vi "Destroy.vi"(8 "error in (no error)":errorcluster, 11 "reference in":refnum<class "Character.lvclass">) -> (0 "error out":errorcluster, 3 "reference out":refnum<class "Character.lvclass">)   [LabVIEW 2012, in "Character.lvclass"]
uses:
  Character.lvclass
  Glyph_class/Glyph.lvclass
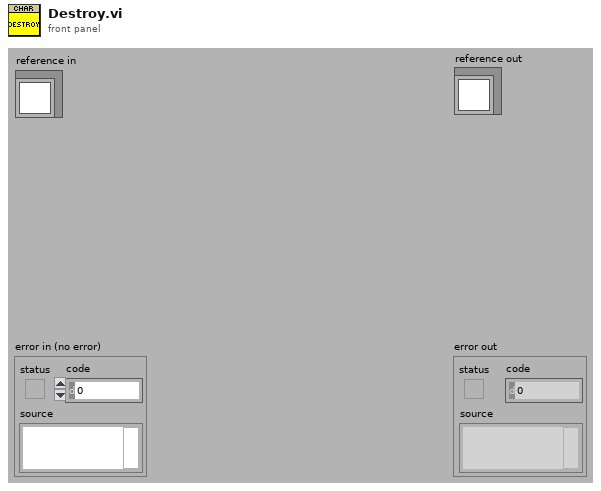
[diagram p1: front panel]
types:
  T1 = typedef "Character.lvclass/ObjectAttributes.ctl" = cluster{"Font":cluster{"Font Name:":string, "Size":i16, "Strikeout?":bool, "Italic?":bool, "Underline?":bool, "Outline?":bool, "Shadow?":bool, "Bold?":bool}, "Color":u32, "Character":string}
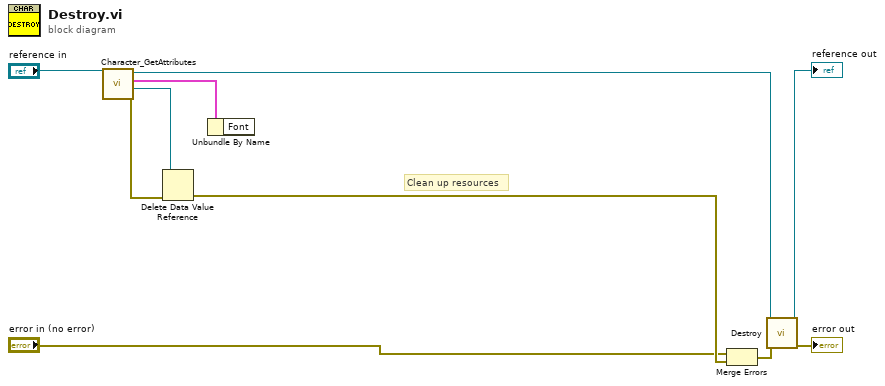
[diagram p0: block diagram]
diagram:
  # "Clean up resources"
  n1 = call "Character_GetAttributes.vi"("reference in"="reference in") -> ("error out"=w9:errorcluster, "DataRef"=w8:refnum<data-value>, "Data"=w7:T1, "reference out"=w4:refnum<class "Character.lvclass">)  [unwired: 7 in]
  n2 = Delete Data Value Reference(data value reference=w8, error in=w9) -> (error out=w6:errorcluster)  [unwired: 1 out]
  n3 = Unbundle By Name(w7) -> ()  [unwired: 1 out]
  n4 = Merge Errors("error in (no error)", w6) -> (w2:errorcluster)
  n5 = call-parent "Destroy.vi"("error in (no error)"=w2, "reference in"=w4) -> ("error out"=→"error out":errorcluster, "reference out"=→"reference out":refnum<class "Character.lvclass">)  [unwired: 8 in]
